vi "CONTROL ARM ANGLE.vi"(0 "refnum name":string="ARMLEFT", 1 "PID gains":T1={"proportional gain (Kc)"=1.0, "integral time (Ti, min)"=0.0, "derivative time (Td, min)"=0.0} {"derivative time (Td, min)" format="%.3f"; "integral time (Ti, min)" format="%.3f"; "proportional gain (Kc)" format="%.6f"}, 2 "output range":cluster{"output high":dbl, "output low":dbl}={"output high"=1.0, "output low"=-1.0} {"output low" format="%.2f"; "output high" format="%.2f"}, 5 "setpoint (in)":dbl(slide) min=-3.5 max=4.5 scale=-3.5..4.5, 7 "error tolerance (in)":dbl=0.0625 format="%#_13g", 9 "times within tolerance":i32=6, 12 "reinitialize? (F)":bool=TRUE, 13 "invert sensor?":bool) -> (8 "position (in)":dbl=-0.056666895292747495, 10 "setpoint error (in)":dbl=0.056666895292747495)   [LabVIEW 2020]
uses:
  Robot Global Data.vi
  <vilib>/Rock Robotics/Network Tables/NT Write Boolean.vi
  <vilib>/addons/control/pid/pid.llb/PID (DBL).vi
  <vilib>/addons/control/pid/NI_PID_pid.lvlib
panel:
  out "x > y?":bool=TRUE
  out "output":dbl=1.0 format="%.2f"
  out "Position":dbl=-1.7619078159332275 format="%.2f"
  out "setpoint 2":dbl
  out "Chart set point & postition 2":cluster{"setpoint":dbl, dbl}(graph)={"setpoint"=0.0, -2.4285731315612793}
  in  "stop":bool
  out "setpoint error (tics)":dbl=2.4285731315612793
  out "Chart motor output":dbl(graph)=1.0
  out "Chart set point & postition":cluster{"setpoint":dbl, dbl}(graph)={"setpoint"=0.0, -0.056666895292747495}
  # "scale 40% @ 2in\n100% @ >5\" error"
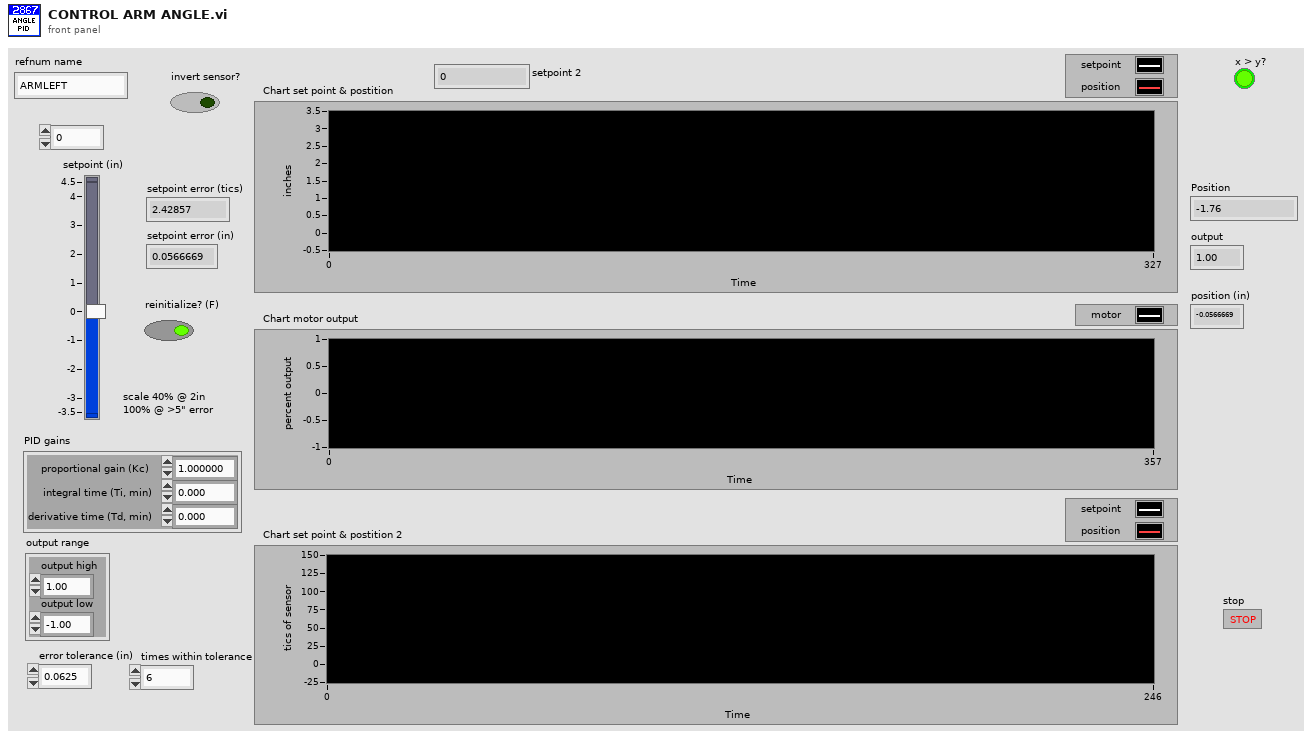
[diagram p1: front panel]
types:
  T1 = cluster{"proportional gain (Kc)":dbl, "integral time (Ti, min)":dbl, "derivative time (Td, min)":dbl}
  T2 = typedef "WPI_MotorControlDeviceRef.ctl" = cluster{"DeviceStatus":errorcluster, "Type":T3, "PWM":cluster{"PWM Channel":T4, "DeadBand":T5}, "CAN":cluster{"Device Number":u8, "SetOutput VI Ref":variant, "GetOutput VI Ref":variant, "Enable VI Ref":variant, "Disable VI Ref":variant, "Data":variant}, "Invert":bool, "DIO PWM":cluster{"PWM \"Enable\" Channel":T4, "DIOChannel":T6, "PWM Rate":dbl}}
  T3 = typedef "WPI_MotorControlType.ctl" = enum16{"PWM", "CAN", "DIO PWM"}
  T4 = typedef "FPGA_DIOPWMChannel.ctl" = enum8{"PWM 0", "PWM 1", "PWM 2", "PWM 3", "PWM 4", "PWM 5", "PWM 6", "PWM 7", "PWM 8", "PWM 9", "PWM MXP 0", "PWM MXP 1", "PWM MXP 2", "PWM MXP 3", "PWM MXP 4", "PWM MXP 5", "PWM MXP 6", "PWM MXP 7", "PWM MXP 8", "PWM MXP 9", "Invalid"}
  T5 = typedef "WPI_PWMDeadband.ctl" = cluster{"Name":string, "maxPositivePwm":i32, "minPositivePwm":i32, "centerPwm":i32, "maxNegativePwm":i32, "minNegativePwm":i32, "angularRange":u16}
  T6 = typedef "FPGA_DIOChannel.ctl" = enum8{"DIO 0", "DIO 1", "DIO 2", "DIO 3", "DIO 4", "DIO 5", "DIO 6", "DIO 7", "DIO 8", "DIO 9", "DIO MXP 0", "DIO MXP 1", "DIO MXP 2", "DIO MXP 3", "DIO MXP 4", "DIO MXP 5", "DIO MXP 6", "DIO MXP 7", "DIO MXP 8", "DIO MXP 9", "DIO MXP 10", "DIO MXP 11", "DIO MXP 12", "DIO MXP 13", "DIO MXP 14", "DIO MXP 15", "SPI Port CS1", "SPI Port CS2", "SPI Port CS3", "SPI Port MISO", "SPI Port MOSI", "Invalid"}
  T7 = cluster{"MIN":dbl, "MAX":dbl, "convert arm inches to revs":dbl, "convert arm inches to degrees":dbl}
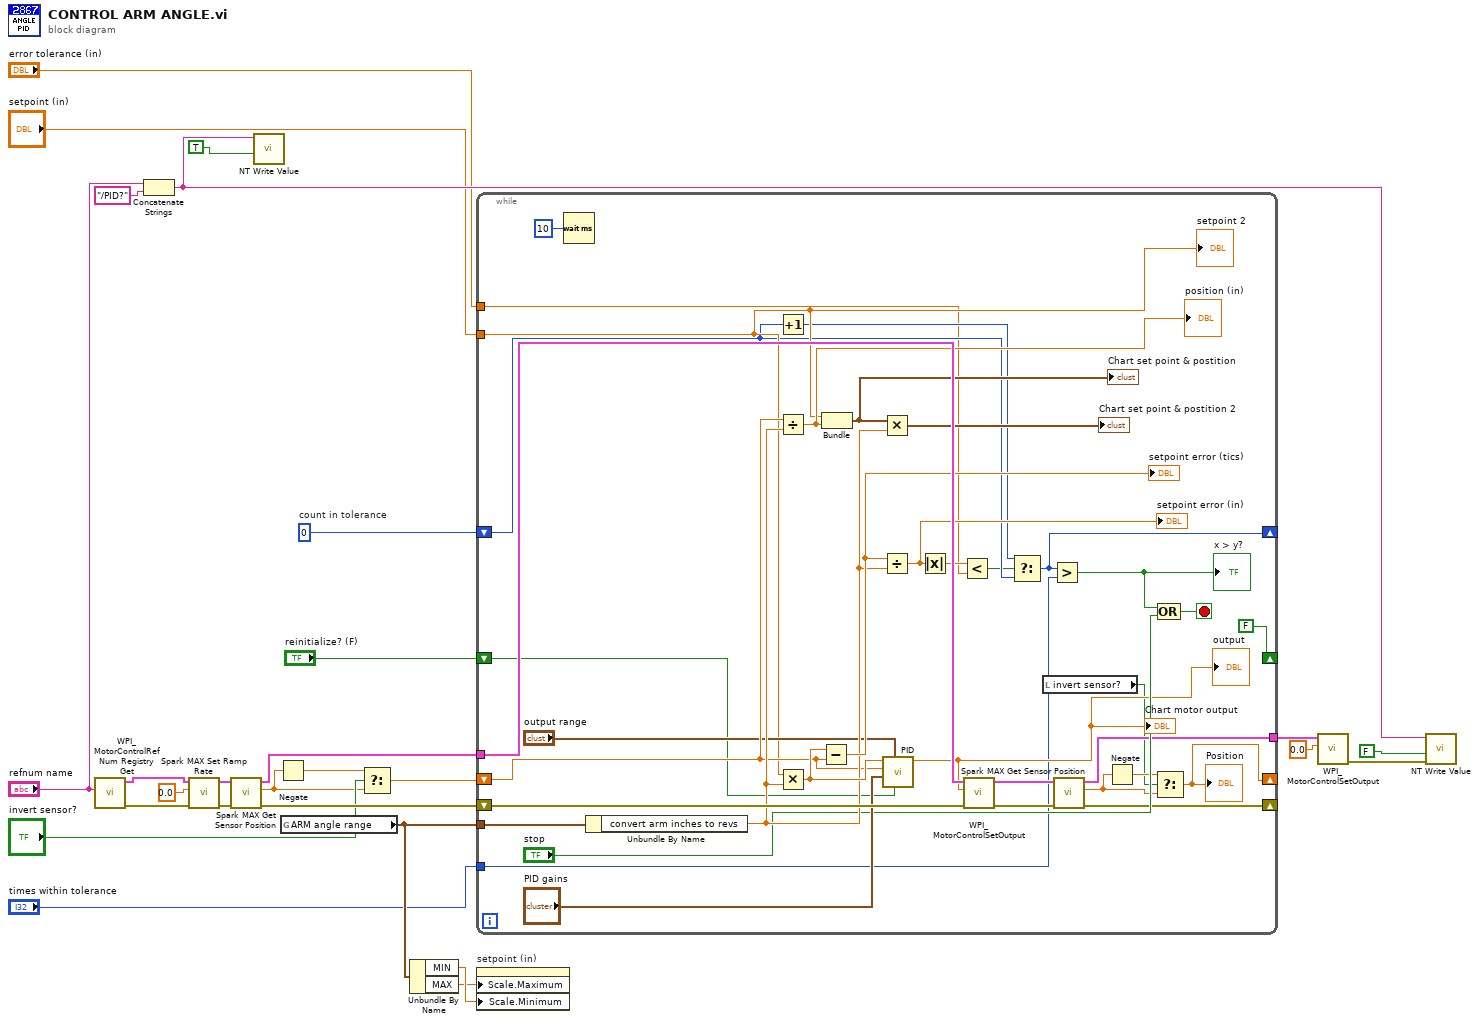
[diagram p0: block diagram]
diagram:
  w8 = 0  # count in tolerance
  n1 = call <vilib>:"WPI_MotorControlRefNum Registry Get.vi"("refnum name"="refnum name") -> ("error out"=w22:errorcluster, "MotorControlDevRef"=w27:T2)  [unwired: 9 in]
  n2 = Concatenate Strings("refnum name", "/PID?" ("string")) -> (w14:string)
  n3 = call <vilib>:"Spark MAX Set Ramp Rate.vi"("error in (no error)"=w22, "Seconds from neutral to full (0)"=0.0 ("secondsFromNeutralToFull"), "MotorControlDeviceRef in"=w27) -> ("error out"=w21:errorcluster, "MotorControlDeviceRef"=w24:T2)  [unwired: 7 in]
  n4 = call <vilib>:"Spark MAX Get Sensor Position.vi"("error in (no error)"=w21, "MotorControlDevRef in"=w24) -> ("error out"=w25:errorcluster, "Sensor Position"=w3:dbl, "MotorControlDevRef out"=w26:T2)  [unwired: 6 in, 1 out]
  n5 = call-poly <vilib>:"NT Write Value.vi"("Boolean"=TRUE, "Name"=w14) -> ()  [unwired: 9 in, 1 out]
  n6 = Negate(x=w3) -> (-x=w2:dbl)
  n7 = global read "Robot Global Data.vi" "ARM angle range"() -> (w20:T7)
  n8 = Select(t=w2, s="invert sensor?", f=w3) -> (s? t:f=w5:dbl)
  n9 = Unbundle By Name(w20) -> ("MIN"=w19:dbl, "MAX"=w18:dbl)
  n10 = while {
    tunnel: w20 -> [w62]
    tunnel: w26 -> [w63]
    shift-right: [w33] -> _
    shift-left: w5 -> [w49]
    shift-right: [w44] -> _
    shift-left: w25 -> [w60]
    tunnel: [w47] -> w13
    tunnel: "setpoint (in)" -> [w43]
    shift-right: [w37] -> _
    shift-left: w8 -> [w40]
    tunnel: "error tolerance (in)" -> [w35]
    tunnel: "times within tolerance" -> [w34]
    shift-right: [FALSE ("reinitialize? (F)")] -> _
    shift-left: "reinitialize? (F)" -> [w29]
    stop <- w50 stop-if-true
    n11 = Wait (ms)(milliseconds to wait=u32 10) -> ()  [unwired: 1 out]
    n12 = Unbundle By Name(w62) -> ("convert arm inches to revs"=w52:dbl)
    n13 = Increment(x=w40) -> (x+1=w38:i32)
    n14 = Divide(x=w49, y=w52) -> (x/y=w55:dbl)
    "position (in)" <- w55
    n15 = Multiply(x=w43, y=w52) -> (x*y=w57:dbl)
    n16 = Subtract(x=w57, y=w49) -> (x-y=w56:dbl)
    "setpoint error (tics)" <- w56
    n17 = Bundle("setpoint (in)"=w43, w55) -> (w54:cluster{"setpoint (in)":dbl, dbl})  [unwired: 1 in]
    "Chart set point & postition" <- w54
    n18 = Multiply(x=w54, y=w52) -> (x*y=→"Chart set point & postition 2":cluster{"setpoint (in)":dbl, dbl})
    n19 = Divide(x=w56, y=w52) -> (x/y=w42:dbl)
    "setpoint error (in)" <- w42
    n20 = call-poly <vilib>:"PID.vi"("reinitialize? (F)"=w29, "output range"="output range", "PID gains"="PID gains", "process variable"=w49, "setpoint"=w57) -> ("output"=w45:dbl)  [unwired: 5 in, 1 out]
    "Chart motor output" <- w45
    "output" <- w45
    n21 = Absolute Value(x=w42) -> (abs(x)=w41:dbl)
    n22 = Less?(x=w41, y=w35) -> (x < y?=w39:bool)
    n23 = call <vilib>:"WPI_MotorControlSetOutput.vi"("error in (no error)"=w60, "Output"=w45, "MotorControlDevRef"=w63) -> ("error out"=w59:errorcluster, "MotorControlDevRef"=w61:T2)  [unwired: 6 in, 1 out]
    n24 = Select(t=w38, s=w39, f=w40) -> (s? t:f=w37:i32)
    n25 = local read "invert sensor?"() -> (w30:bool)
    n26 = Greater?(x=w37, y=w34) -> (0:w36:bool)
    "x > y?" <- w36
    n27 = call <vilib>:"Spark MAX Get Sensor Position.vi"("error in (no error)"=w59, "MotorControlDevRef in"=w61) -> ("error out"=w44:errorcluster, "Sensor Position"=w32:dbl, "MotorControlDevRef out"=w47:T2)  [unwired: 6 in, 1 out]
    n28 = Negate(x=w32) -> (-x=w31:dbl)
    n29 = Select(t=w31, s=w30, f=w32) -> (s? t:f=w33:dbl)
    "Position" <- w33
    n30 = Compound Arithmetic op=OR(w36, "stop") -> (w50:bool)
    "setpoint 2" <- w43
  }
  n31 = property on="setpoint (in)" class="Slide (strict)"("Scale.Maximum"=w18, "Scale.Minimum"=w19) -> ()  [unwired: 2 in, 2 out]
  n32 = call <vilib>:"WPI_MotorControlSetOutput.vi"("Output"=0.0, "MotorControlDevRef"=w13) -> ("error out"=w10:errorcluster)  [unwired: 7 in, 2 out]
  n33 = call-poly <vilib>:"NT Write Value.vi"("error in"=w10, "Boolean"=FALSE, "Name"=w14) -> ()  [unwired: 8 in, 1 out]
